vi "newRampTime.vi"(8 "error in (no error)":errorcluster, 11 "RampAction in":refnum<class "RampAction.lvclass">) -> (0 "error out":errorcluster, 3 "RampAction out":refnum<class "RampAction.lvclass">)   [LabVIEW 2011, in "Views.lvlib" / "ScriptEditor.lvlib" / "RampAction.lvclass"]
uses:
  RampAction.lvclass
  RampAction.lvclass/RampAction.ctl
  Tools/Scripting/ScriptingEvent/ScriptEvents/Ramp/RampEvent/RampEvent.lvclass
  ActionPanel.lvclass
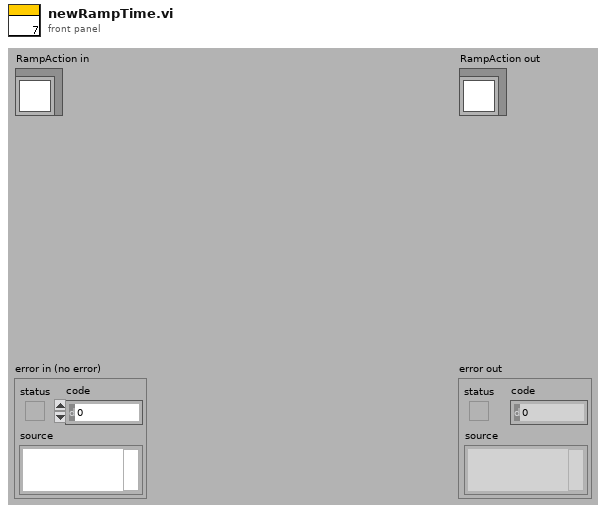
[diagram p1: front panel]
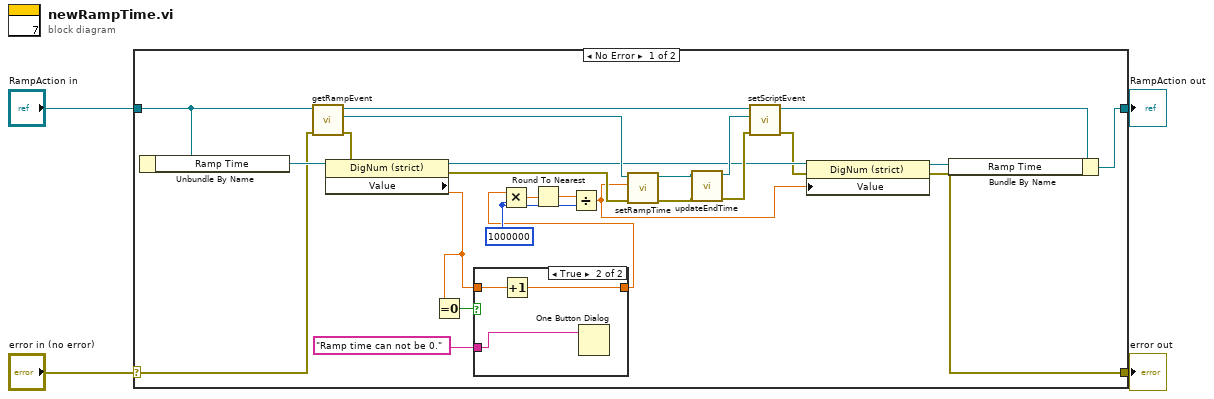
[diagram p0: block diagram]
diagram:
  n1 = case shown="No Error" "error in (no error)" {
    selector: "error in (no error)" -> [w23 w35]
    tunnel: [w8 w35] -> w3
    tunnel: [w6 w34] -> w1
    tunnel: "RampAction in" -> [w28 w34]
    frame No Error {
      w16 = 1000000
      n2 = Unbundle By Name(w28) -> ("Ramp Time"=w29:refnum<vi>)
      n3 = call "getRampEvent.vi"("error in (no error)"=w23, "RampAction in"=w28) -> ("error out"=w27:errorcluster, "RampEvent"=w26:refnum<class "RampEvent.lvclass">, "RampAction out"=w24:refnum<class "RampAction.lvclass">)  [unwired: 7 in]
      n4 = property class="DigNum (strict)"(reference=w29, error in=w27) -> (reference out=w12:refnum<vi>, error out=w25:errorcluster, "Value"=w14:dbl)
      n5 = Equal To 0?(x=w14) -> (x = 0?=w13:bool)
      n6 = case shown="True" w13 {
        tunnel: [w30 w33] -> w11
        tunnel: "Ramp time can not be 0." -> [_ w32]
        tunnel: w14 -> [w30 w31]
        frame False {
        }
        frame True {
          n7 = Increment(x=w31) -> (x+1=w33:dbl)
          n8 = One Button Dialog(message=w32) -> ()  [unwired: 1 in, 1 out]
        }
      }
      n9 = Multiply(x=w11, y=w16) -> (x*y=w18:dbl)
      n10 = Round To Nearest(number=w18) -> (nearest integer value=w17:dbl)
      n11 = Divide(x=w17, y=w16) -> (x/y=w10:dbl)
      n12 = call "setRampTime.vi"("error in (no error)"=w25, "rampTime"=w10, "RampEvent.lvclass in"=w26) -> ("error out"=w21:errorcluster, "RampEvent.lvclass out"=w22:refnum<class "RampEvent.lvclass">)  [unwired: 7 in]
      n13 = call-dynamic "updateEndTime.vi"("error in (no error)"=w21, "RampEvent in"=w22) -> ("error out"=w20:errorcluster, "RampEvent out"=w19:refnum<class "RampEvent.lvclass">)  [unwired: 8 in]
      n14 = call "setScriptEvent.vi"("error in (no error)"=w20, "ScriptEvent.lvclass"=w19, "ActionPanel.lvclass in"=w24) -> ("error out"=w9:errorcluster, "ActionPanel.lvclass out"=w7:refnum<class "RampAction.lvclass">)  [unwired: 7 in]
      n15 = property class="DigNum (strict)"(reference=w12, error in=w9, "Value"=w10) -> (reference out=w5:refnum<vi>, error out=w8:errorcluster)
      n16 = Bundle By Name(cluster=w7, "Ramp Time"=w5) -> (w6:refnum<class "RampAction.lvclass">)
    }
    frame Error {
    }
  }
  "error out" <- w3
  "RampAction out" <- w1
